vi "tc_status.vi"(8 "Numeric":dbl, 9 "reference":refnum<vi>, 10 "Boolean":bool, 11 "Digital in":refnum<vi>) -> ()   [LabVIEW 2017]
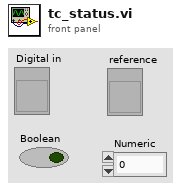
[diagram p1: front panel]
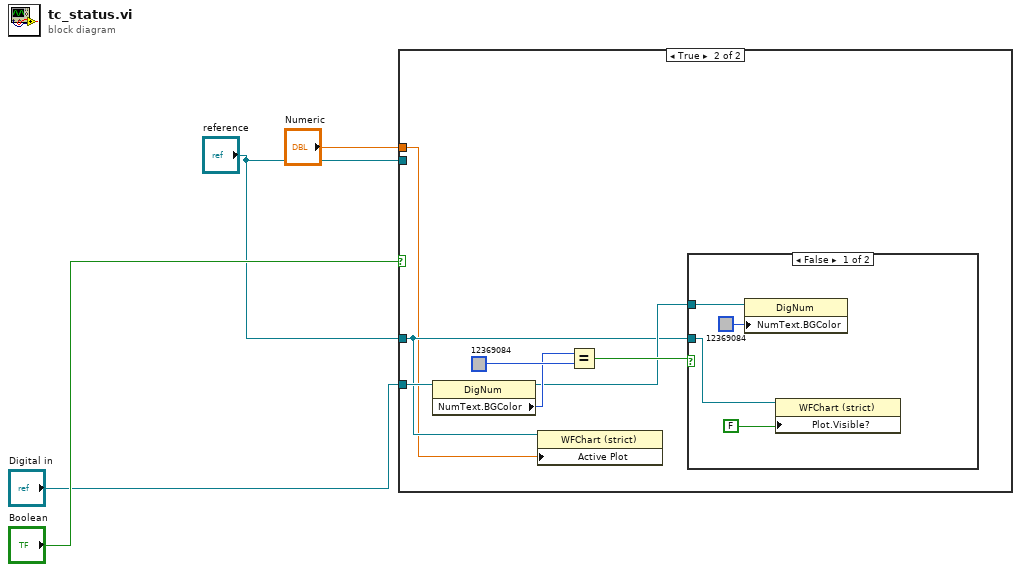
[diagram p0: block diagram]
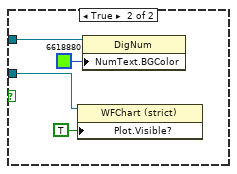
[diagram p3: hidden frame]
diagram:
  n1 = case shown="True" "Boolean" {
    tunnel: "Digital in" -> [_ w9]
    tunnel: "reference" -> [_ _]
    tunnel: "reference" -> [_ w6]
    tunnel: "Numeric" -> [_ w5]
    frame False {
    }
    frame True {
      n2 = property class="DigNum"(reference=w9) -> (reference out=w7:refnum<vi>, "NumText.BGColor"=w8:u32)  [unwired: 1 in, 1 out]
      n3 = property class="WFChart (strict)"(reference=w6, "Active Plot"=w5) -> ()  [unwired: 1 in, 2 out]
      n4 = Equal?(x=w8, y=u32 12369084) -> (x = y?=w10:bool)
      n5 = case shown="False" w10 {
        tunnel: w7 -> [w14 w18]
        tunnel: w6 -> [w12 w16]
        frame False {
          n6 = property class="DigNum"(reference=w14, "NumText.BGColor"=u32 12369084) -> ()  [unwired: 1 in, 2 out]
          n7 = property on="Property Node" class="WFChart (strict)"(reference=w12, "Plot.Visible?"=FALSE ("Plot.Visible")) -> ()  [unwired: 1 in, 2 out]
        }
        frame True {
          n8 = property on="Property Node" class="WFChart (strict)"(reference=w16, "Plot.Visible?"=TRUE ("Plot.Visible")) -> ()  [unwired: 1 in, 2 out]
          n9 = property class="DigNum"(reference=w18, "NumText.BGColor"=u32 6618880) -> ()  [unwired: 1 in, 2 out]
        }
      }
    }
  }
